vi "Read Prepend Result Name.vi"(8 "error in (no error)":errorcluster, 11 "SeqAuto IEvaluation in":refnum<class "SeqAuto IEvaluation.lvclass">) -> (0 "error out":errorcluster, 2 "Prepend Result Name":bool, 3 "SeqAuto IEvaluation out":refnum<class "SeqAuto IEvaluation.lvclass">)   [LabVIEW 2018, in "IEvaluation.lvlib" / "SeqAuto IEvaluation.lvclass"]
uses:
  SeqAuto IEvaluation.lvclass
  SeqAuto IEvaluation.lvclass/SeqAuto IEvaluation.ctl
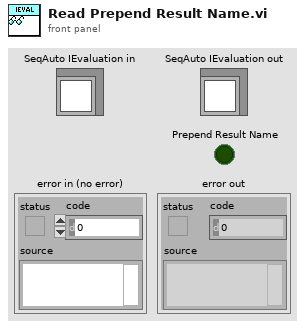
[diagram p1: front panel]
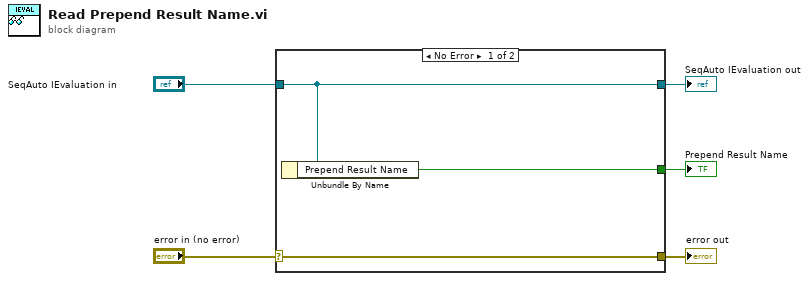
[diagram p0: block diagram]
diagram:
  n1 = case shown="No Error" "error in (no error)" {
    selector: "error in (no error)" -> [w8 w9]
    tunnel: [w8 w9] -> w4
    tunnel: [w7 w10] -> w2
    tunnel: "SeqAuto IEvaluation in" -> [w7 w10]
    tunnel: [w6 _] -> w1
    frame No Error {
      n2 = Unbundle By Name(w7) -> ("Prepend Result Name"=w6:bool)
    }
    frame Error {
    }
  }
  "error out" <- w4
  "SeqAuto IEvaluation out" <- w2
  "Prepend Result Name" <- w1
